vi "fgv_F9P_data.vi"(7 "cmd":T2, 11 "ublox UBX data":T1) -> ()   [LabVIEW 2019]
uses:
  Ctrl/cmd_common.ctl
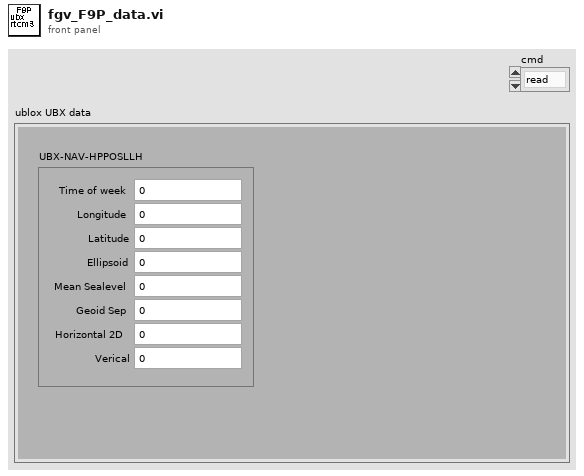
[diagram p1: front panel]
types:
  T1 = cluster{"UBX-NAV-HPPOSLLH":cluster{"Time of week":dbl, "Longitude":dbl, "Latitude":dbl, "Ellipsoid":dbl, "Mean Sealevel":dbl, "Geoid Sep":dbl, "Horizontal 2D":dbl, "Verical":dbl}}
  T2 = typedef "cmd_common.ctl" = enum16{"read", "write"}
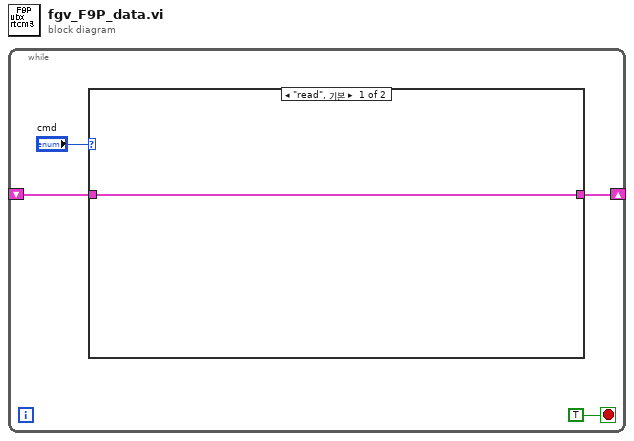
[diagram p0: block diagram]
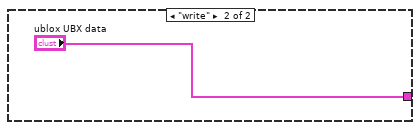
[diagram p2: hidden frame]
diagram:
  n1 = while {
    shift-right: [w2] -> _
    shift-left: _ -> [w1]
    stop <- TRUE stop-if-true
    n2 = case shown="\"read\", 기본" "cmd" {
      tunnel: [w5 "ublox UBX data"] -> w2
      tunnel: w1 -> [w5 _]
      frame "read", Default {
      }
      frame "write" {
      }
    }
  }
